vi "List VIs without Test Coverage.vi"(8 "error in (no error)":errorcluster, 9 "Tests Root":path, 10 "Source Root":path, 11 "Project Root":path) -> (0 "error out":errorcluster, 1 "Test VIs":path[](array[path]), 2 "VIs without test coverage":string[](array[string]), 3 "coverage.json":string)   [LabVIEW 2020]
panel:
  out "coverage.txt":string
  out "source VIs":string[](array[string])
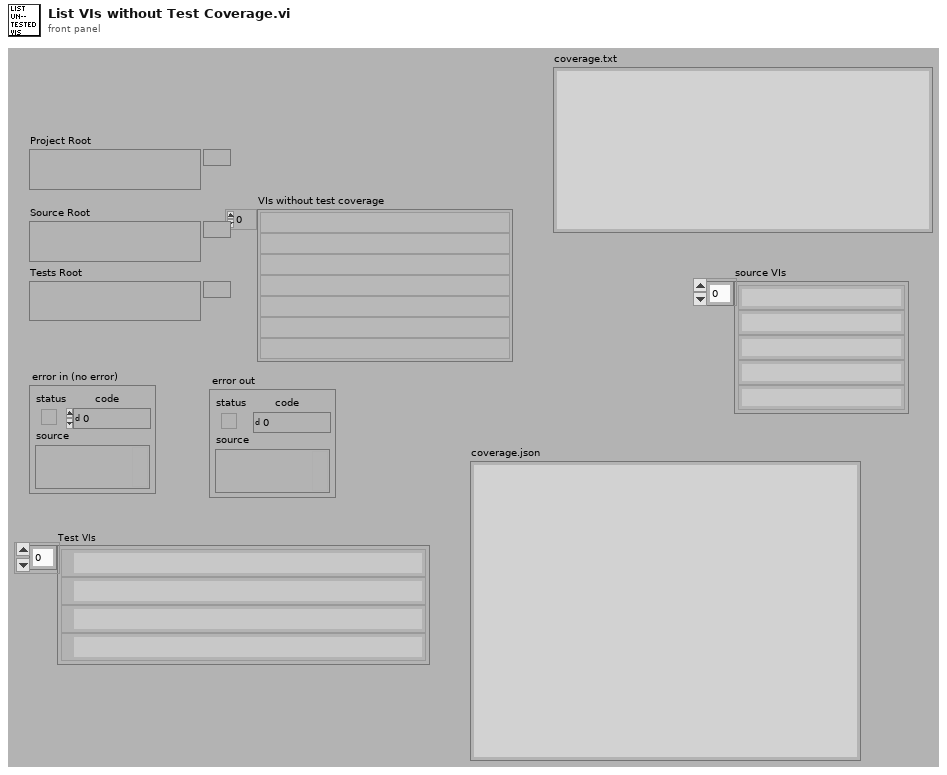
[diagram p1: front panel]
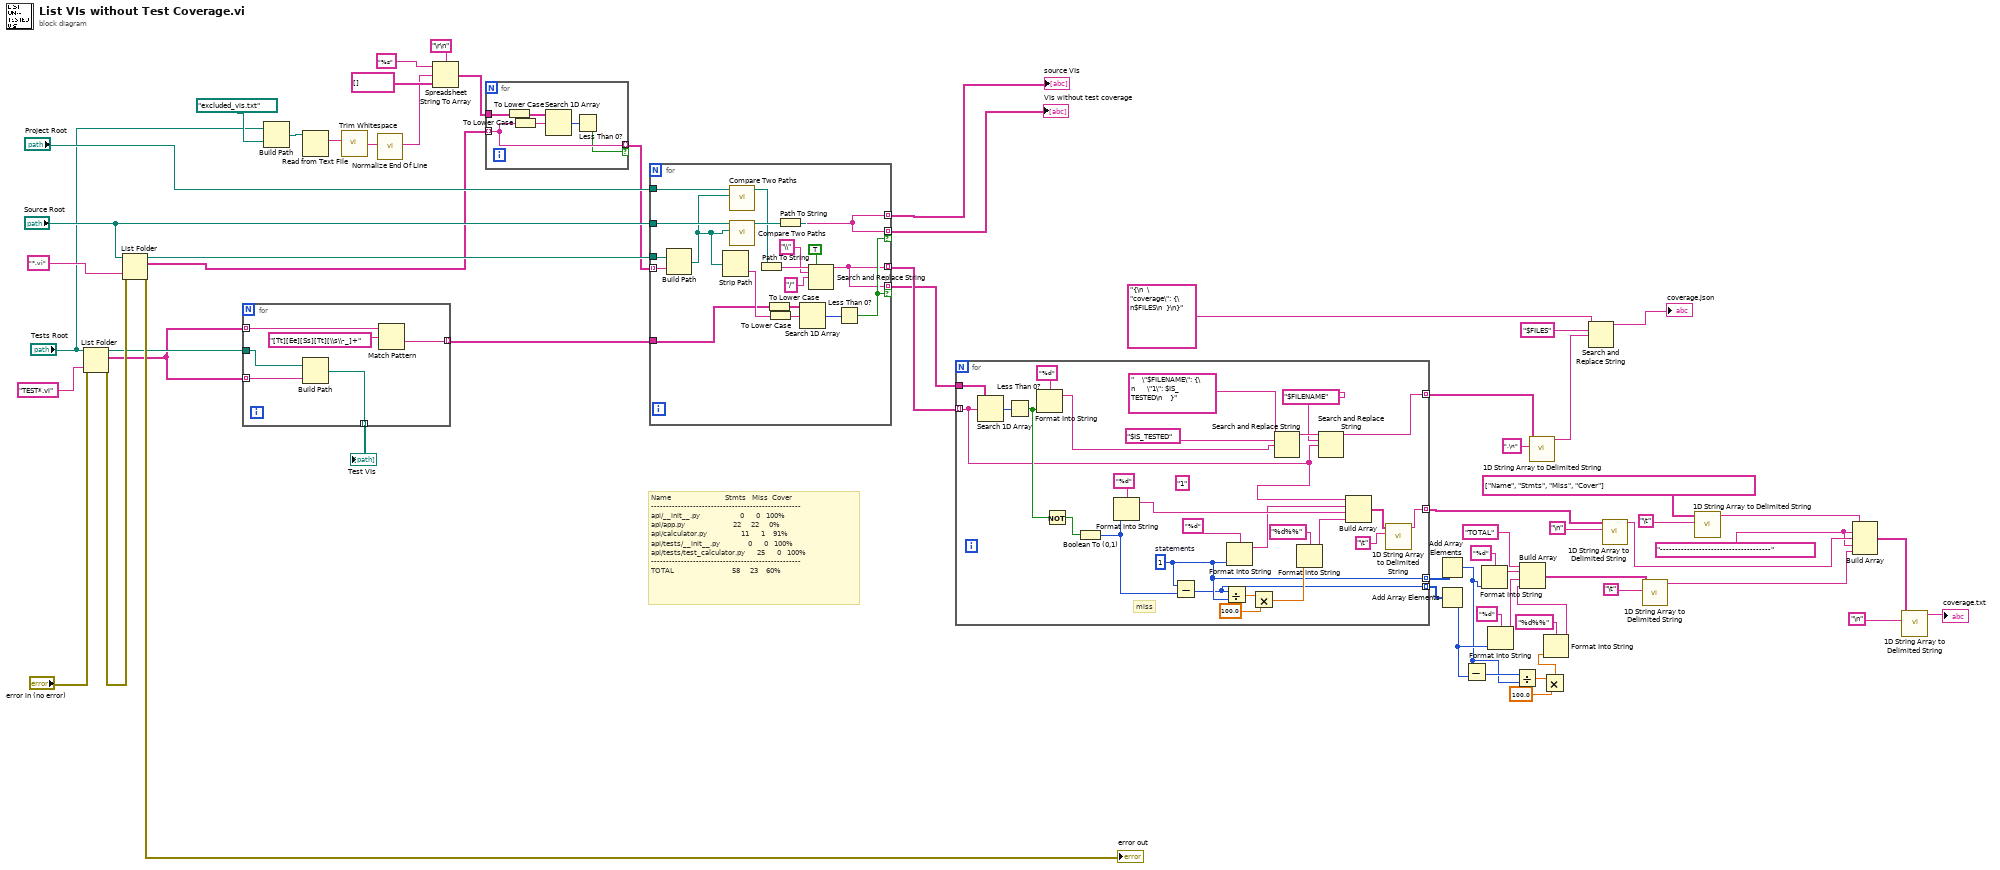
[diagram p0: block diagram]
diagram:
  w18 = "-------------------------------------"
  # "Name                           Stmts   Miss  Cover\n--------------------------------------------------\napi/__init__.py                    0      0   100%\napi/app.py                        22     22     0%\napi/calculator.py                 11      1    91%\napi/tests/__init__.py              0      0   100%\napi/tests/test_calculator.py      25      0   100%\n--------------------------------------------------\nTOTAL                             58     23    60%"
  n1 = List Folder(path="Tests Root", pattern="TEST*.vi", error in="error in (no error)") -> (path out=w54:path, filenames=w53:string[], error out=w60:errorcluster)  [unwired: 1 in, 1 out]
  n2 = List Folder(path="Source Root", pattern="*.vi", error in=w60) -> (path out=w55:path, filenames=w2:string[], error out=→"error out":errorcluster)  [unwired: 1 in, 1 out]
  n3 = for {
    tunnel: w53 -> [w68] mode=indexing
    tunnel: [w66] -> w59 mode=indexing
    tunnel: w54 -> [w65]
    tunnel: w53 -> [w64] mode=indexing
    tunnel: [w63] -> w52 mode=indexing
    n4 = Build Path(base path=w65, name or relative path=w64) -> (appended path=w63:path)
    n5 = Match Pattern(string=w68, regular expression="[Tt][Ee][Ss][Tt][\\s\\-_]+") -> (after substring=w66:string)  [unwired: 1 in, 3 out]
  }
  "Test VIs" <- w52
  n6 = Build Path(base path="Tests Root", name or relative path=path "excluded_vis.txt" ("Relative path (.)")) -> (appended path=w11:path)
  n7 = Read from Text File(file (use dialog)=w11) -> (text=w5:string)  [unwired: 3 in, 3 out]
  n8 = call <vilib>:"Trim Whitespace.vi"("string"=w5) -> ("trimmed string"=w7:string)  [unwired: 1 in]
  n9 = call <vilib>:"Normalize End Of Line.vi"("string in"=w7) -> ("string out"=w6:string)  [unwired: 7 in]
  n10 = Spreadsheet String To Array(delimiter (Tab)="\r\n", format string="%s", spreadsheet string=w6, array type (2D Dbl)=string[] [] ("appended array")) -> (array=w3:string[])
  n11 = for {
    tunnel: w2 -> [w72] mode=indexing
    tunnel: w3 -> [w74]
    tunnel: [w72] -> w1 mode=indexing if=w71
    n12 = To Lower Case(string=w74) -> (all lower case string=w69:string[])
    n13 = To Lower Case(string=w72) -> (all lower case string=w70:string)
    n14 = Search 1D Array(1D array=w69, element=w70) -> (index of element=w73:i32)  [unwired: 1 in]
    n15 = Less Than 0?(x=w73) -> (x < 0?=w71:bool)
  }
  n16 = for {
    tunnel: w59 -> [w92]
    tunnel: "Source Root" -> [w88]
    tunnel: [w84] -> w42 mode=indexing if=w80
    tunnel: w55 -> [w90]
    tunnel: w1 -> [w89] mode=indexing
    tunnel: [w84] -> w44 mode=indexing
    tunnel: "Project Root" -> [w83]
    tunnel: [w78] -> w43 mode=indexing
    tunnel: [w78] -> w41 mode=indexing if=w80
    n17 = Build Path(base path=w90, name or relative path=w89) -> (appended path=w82:path)
    n18 = Strip Path(path=w82) -> (name=w93:string)  [unwired: 1 out]
    n19 = call <vilib>:"Compare Two Paths.vi"("Path 2"=w82, "Path 1"=w83) -> ("Relative Path from 1 to 2"=w81:path)  [unwired: 6 in, 3 out]
    n20 = call <vilib>:"Compare Two Paths.vi"("Path 2"=w82, "Path 1"=w88) -> ("Relative Path from 1 to 2"=w85:path)  [unwired: 6 in, 3 out]
    n21 = Path To String(path=w81) -> (string=w79:string)
    n22 = To Lower Case(string=w92) -> (all lower case string=w86:string[])
    n23 = To Lower Case(string=w93) -> (all lower case string=w87:string)
    n24 = Path To String(path=w85) -> (string=w84:string)
    n25 = Search 1D Array(1D array=w86, element=w87) -> (index of element=w91:i32)  [unwired: 1 in]
    n26 = Search and Replace String(replace all?=TRUE ("replace all? (F)"), input string=w79, search string="\\", replace string="/" ("search string")) -> (result string=w78:string)  [unwired: 4 in, 3 out]
    n27 = Less Than 0?(x=w91) -> (x < 0?=w80:bool)
  }
  "VIs without test coverage" <- w42
  "source VIs" <- w44
  n28 = for {
    tunnel: [w113] -> w48 mode=indexing
    tunnel: w43 -> [w108] mode=indexing
    tunnel: w41 -> [w118]
    tunnel: [w94] -> w24 mode=indexing
    tunnel: [w98] -> w40 mode=indexing
    tunnel: [w97] -> w39 mode=indexing
    w98 = 1  # statements
    (unwired) "1"
    # "miss"
    n29 = Search 1D Array(1D array=w118, element=w108) -> (index of element=w117:i32)  [unwired: 1 in]
    n30 = Less Than 0?(x=w117) -> (x < 0?=w111:bool)
    n31 = Format Into String(format string="%d", w111) -> (resulting string=w115:string)  [unwired: 2 in, 1 out]
    n32 = Not(x=w111) -> (.not. x?=w107:bool)
    n33 = Boolean To (0,1)(Boolean=w107) -> (0, 1=w104:i16)
    n34 = Format Into String(format string="%d", w104) -> (resulting string=w109:string)  [unwired: 2 in, 1 out]
    n35 = Subtract(x=w98, y=w104) -> (x-y=w97:i32)
    n36 = Divide(x=w97, y=w98) -> (x/y=w103:dbl)
    n37 = Format Into String(format string="%d", w98) -> (resulting string=w105:string)  [unwired: 2 in, 1 out]
    n38 = Multiply(x=w103, y=100.0) -> (x*y=w100:dbl)
    n39 = Search and Replace String(input string="    \"$FILENAME\": {\n      \"1\": $IS_TESTED\n    }", search string="$IS_TESTED" ("delimiter"), replace string=w115) -> (result string=w114:string)  [unwired: 5 in, 3 out]
    n40 = Format Into String(format string="%d%%", w100) -> (resulting string=w101:string)  [unwired: 2 in, 1 out]
    n41 = Search and Replace String(input string=w114, search string="$FILENAME" ("delimiter"), replace string=w108) -> (result string=w113:string)  [unwired: 5 in, 3 out]
    n42 = Build Array(w108, w105, w109, w101) -> (w95:string[])
    n43 = call <vilib>:"1D String Array to Delimited String.vi"("delimiter"="\t", "string array"=w95) -> ("delimited string"=w94:string)  [unwired: 9 in]
  }
  n44 = Add Array Elements(numeric array=w40) -> (sum=w13:i32)
  n45 = Add Array Elements(numeric array=w39) -> (sum=w30:i32)
  n46 = Subtract(x=w13, y=w30) -> (x-y=w33:i32)
  n47 = Format Into String(format string="%d", w13) -> (resulting string=w38:string)  [unwired: 2 in, 1 out]
  n48 = Format Into String(format string="%d", w30) -> (resulting string=w35:string)  [unwired: 2 in, 1 out]
  n49 = Divide(x=w33, y=w13) -> (x/y=w31:dbl)
  n50 = call <vilib>:"1D String Array to Delimited String.vi"("delimiter"=",\n", "string array"=w48) -> ("delimited string"=w47:string)  [unwired: 9 in]
  n51 = Multiply(x=w31, y=100.0) -> (x*y=w28:dbl)
  n52 = Format Into String(format string="%d%%", w28) -> (resulting string=w27:string)  [unwired: 2 in, 1 out]
  n53 = Build Array("TOTAL", w38, w35, w27) -> (w21:string[])
  n54 = Search and Replace String(input string="{\n  \"coverage\": {\n$FILES\n  }\n}", search string="$FILES", replace string=w47) -> (result string=→"coverage.json":string)  [unwired: 5 in, 3 out]
  n55 = call <vilib>:"1D String Array to Delimited String.vi"("delimiter"="\n", "string array"=w24) -> ("delimited string"=w19:string)  [unwired: 9 in]
  n56 = call <vilib>:"1D String Array to Delimited String.vi"("delimiter"="\t", "string array"=w21) -> ("delimited string"=w17:string)  [unwired: 9 in]
  n57 = call <vilib>:"1D String Array to Delimited String.vi"("delimiter"="\t", "string array"=string[] ["Name", "Stmts", "Miss", "Cover"]) -> ("delimited string"=w20:string)  [unwired: 9 in]
  n58 = Build Array(w20, w18, w19, w18, w17) -> (w15:string[])
  n59 = call <vilib>:"1D String Array to Delimited String.vi"("delimiter"="\n", "string array"=w15) -> ("delimited string"=→"coverage.txt":string)  [unwired: 9 in]
